vi "ConnectionStatus.vi"(10 "Camera_status":bool, 11 "cDAQ_status":bool) -> (0 "String":string="Connections: Terminate\nConnections: Initialize", 3 "SystemStatus":bool)   [LabVIEW 2020]
panel:
  in  "Connect":bool
  out "Cam":bool
  out "cDAQ":bool
  in  "OK":bool
  # "cDAQ"
  # "Camera"
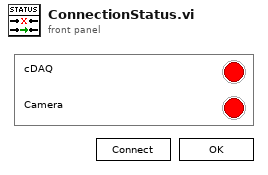
[diagram p1: front panel]
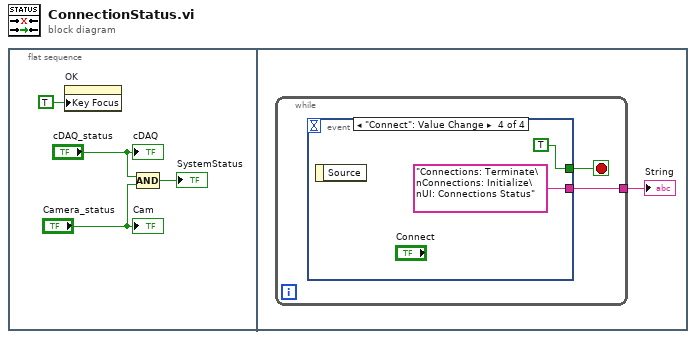
[diagram p0: block diagram]
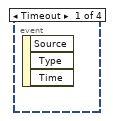
[diagram p2: hidden frame]
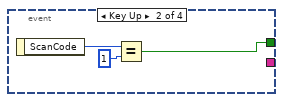
[diagram p3: hidden frame]
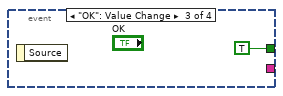
[diagram p4: hidden frame]
diagram:
  n1 = flat-sequence {
    frame #0 {
      n2 = property on="OK" class="Bool"("Key Focus"=TRUE) -> ()  [unwired: 2 in, 2 out]
      n3 = Compound Arithmetic op=AND("cDAQ_status", "Camera_status") -> (→"SystemStatus":bool)
      "cDAQ" <- "cDAQ_status"
      "Cam" <- "Camera_status"
    }
    frame #1 {
      n4 = while {
        tunnel: [w6] -> w5
        stop <- w7 stop-if-true
        n5 = event shown="[3] \"Connect\": Value Change" {
          selector: _ -> [_ _ _ _]
          dyn-events: _ -> [_ _ _ _]
          timeout: _ -> [_ _ _ _]
          tunnel: [_ w8 TRUE TRUE] -> w7
          tunnel: [_ _ _ "Connections: Terminate\nConnections: Initialize\nUI: Connections Status"] -> w6
          event Timeout {
            n6 = event-data() -> ()  [unwired: 1 in, 3 out]
          }
          event Key Up {
            n7 = event-data() -> ("ScanCode"=w10:i16)  [unwired: 1 in]
            n8 = Equal?(x=w10, y=i16 1) -> (x = y?=w8:bool)
          }
          event "OK": Value Change {
            n9 = event-data() -> ()  [unwired: 1 in, 1 out]
          }
          event "Connect": Value Change {
            n10 = event-data() -> ()  [unwired: 1 in, 1 out]
          }
        }
      }
      "String" <- w5
    }
  }
